vi "KE622x -- Get Filter Params.vi"(0 "Resource In":refnum<visa-resource-name>, 1 "Check For SCPI Errors? (T)":bool=TRUE, 11 "error in (no error)":errorcluster) -> (4 "Resource Out (dupl)":refnum<visa-resource-name>, 8 "Filter Params":T1={"Filter Enabled?"=TRUE, "Filter Type"=enum."Moving Ave", "Filter Length"=10, "Filter Window (%)"=0.0} {"Filter Window (%)" min=0.0 max=10.0 step=0.01 format="%.2f"; "Filter Length" min=2 max=300}, 15 "error out":errorcluster)   [LabVIEW 2019, in "Keithley 622x.lvlib"]
doc: "Returns the parameters of the digital filter in the instrument, and also whether or not the filter is enabled. Note that since the 622x instrument doesn't really make any measurements, use of the digital implies that the 622x is being used in conjunction with a 2182/2182A nano-voltmeter."
uses:
  Keithley 622x.lvlib
  Typedefs/KE622x -- Filter Params.ctl
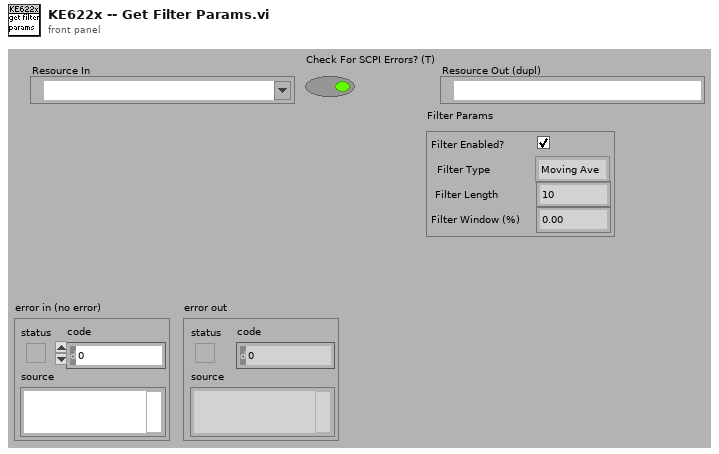
[diagram p1: front panel]
types:
  T1 = typedef "Keithley 622x.lvlib/KE622x -- Filter Params.ctl" = cluster{"Filter Enabled?":bool, "Filter Type":enum16{"Moving Ave", "Repeat Ave"}, "Filter Length":u32, "Filter Window (%)":dbl}
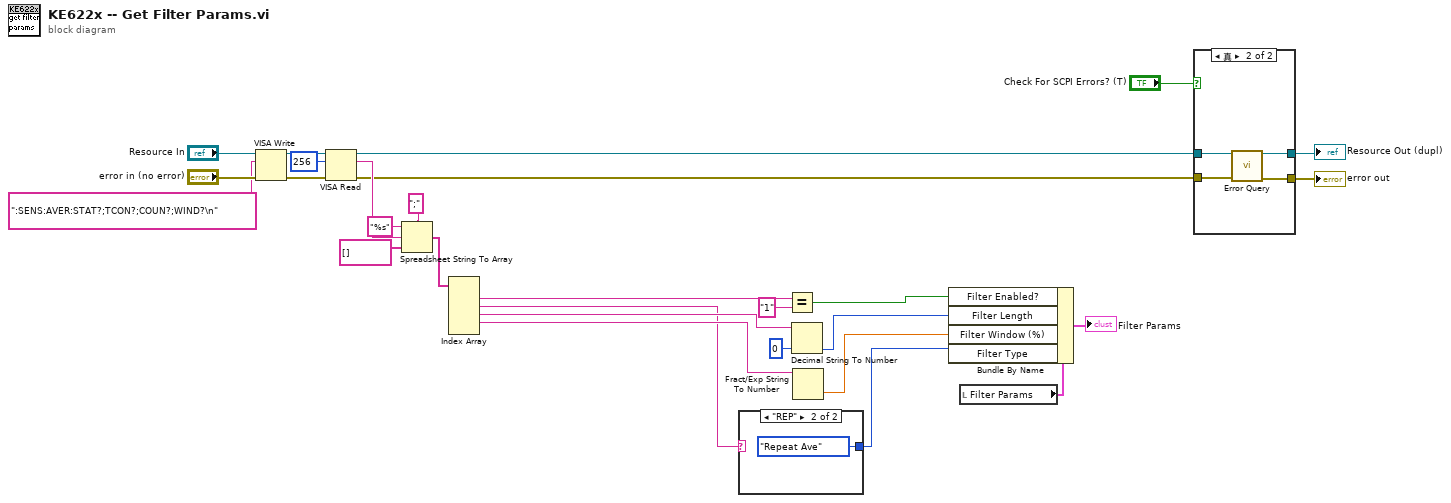
[diagram p0: block diagram]
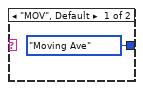
[diagram p2: hidden frame]
diagram:
  n1 = VISA Write(VISA resource name="Resource In", write buffer=":SENS:AVER:STAT?;TCON?;COUN?;WIND?\n" ("format string"), error in (no error)="error in (no error)") -> (VISA resource name out=w22:refnum<visa-resource-name>, error out=w21:errorcluster)  [unwired: 1 out]
  n2 = VISA Read(VISA resource name=w22, byte count=u32 256, error in (no error)=w21) -> (VISA resource name out=w19:refnum<visa-resource-name>, read buffer=w18:string, error out=w2:errorcluster)  [unwired: 1 out]
  n3 = Spreadsheet String To Array(delimiter (Tab)=";", format string="%s", spreadsheet string=w18, array type (2D Dbl)=string[] []) -> (array=w14:string[])
  n4 = Index Array(array=w14) -> (element #1=w13:string, element #2=w3:string, element #3=w8:string, element #4=w5:string)  [unwired: 5 in, 1 out]
  n5 = case shown="\"REP\"" w3 {
    tunnel: [enum16{"Moving Ave", "Repeat Ave"}."Moving Ave" ("Filter Type") enum16{"Moving Ave", "Repeat Ave"}."Repeat Ave" ("Filter Type")] -> w1
    frame "MOV", Default {
    }
    frame "REP" {
    }
  }
  n6 = Equal?(x=w13, y="1") -> (x = y?=w10:bool)
  n7 = Decimal String To Number(string=w8, default (0L)=u32 0 ("default (0 I32)")) -> (number=w7:u32)  [unwired: 1 in, 1 out]
  n8 = Fract/Exp String To Number(string=w5) -> (number=w4:dbl)  [unwired: 3 in, 1 out]
  n9 = local read "Filter Params"() -> (w11:T1)
  n10 = Bundle By Name(cluster=w11, "Filter Enabled?"=w10, "Filter Length"=w7, "Filter Window (%)"=w4, "Filter Type"=w1) -> (→"Filter Params":T1)
  n11 = case shown="真" "Check For SCPI Errors? (T)" {
    tunnel: w19 -> [w32 w36]
    tunnel: [w31 w35] -> w24
    tunnel: [w32 w34] -> w25
    tunnel: w2 -> [w31 w33]
    frame False {
    }
    frame True {
      n12 = call "Error Query.vi"("VISA Resource In"=w36, "error in (no error)"=w33) -> ("VISA Resource Out (dupl)"=w34:refnum<visa-resource-name>, "error out"=w35:errorcluster)  [unwired: 10 in, 2 out]
    }
  }
  "Resource Out (dupl)" <- w25
  "error out" <- w24
